vi "Test MinMax Decimation.vi"() -> ()   [LabVIEW 2020, in "VolatusScratch.lvlib"]
uses:
  VolatusScratch.lvlib
  VolatusGUIElements/VolatusGUIElements.lvlib
  <vilib>/Analysis/NI_AALBase.lvlib
panel:
  in  "Width":dbl=20.0 format="%#_13g"
  in  "Length s":dbl=10.0 format="%#_13g"
  out "XY Graph":cluster{dbl[], "Sinusoidal Pattern":dbl[]}[](graph)
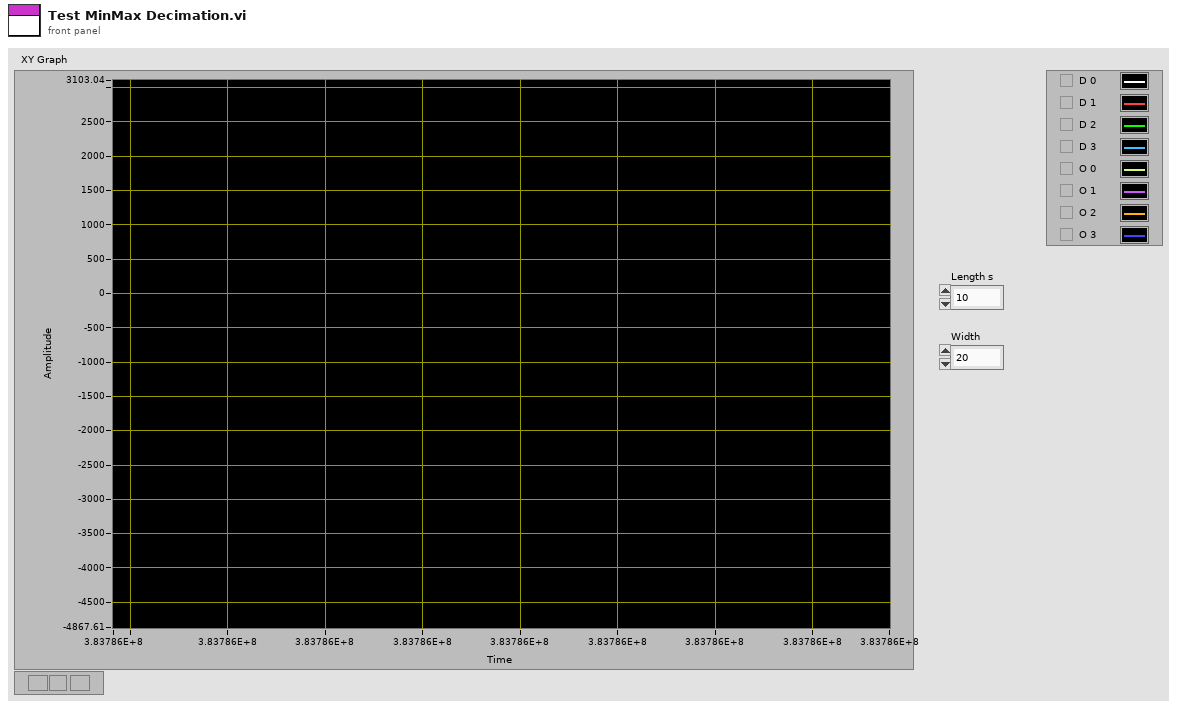
[diagram p1: front panel]
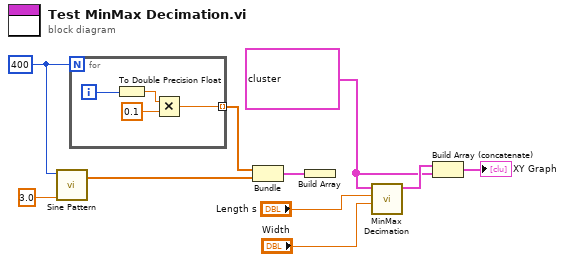
[diagram p0: block diagram]
diagram:
  w1 = cluster{dbl[], "Sinusoidal Pattern":dbl[]}[] [{array[5416 elements], "Sinusoidal Pattern"=array[5416 elements]}, {array[5416 elements], "Sinusoidal Pattern"=array[5416 elements]}, {array[5416 elements], "Sinusoidal Pattern"=array[5416 elements]}, {array[5416 elements], "Sinusoidal Pattern"=array[5416 elements]}] ("appended array")
  w7 = 400 ("samples")
  n1 = call <vilib>:"Sine Pattern.vi"("cycles"=3.0, "samples"=w7) -> ("Sinusoidal Pattern"=w6:dbl[])  [unwired: 2 in, 1 out]
  n2 = for {
    N: w7 -> [_]
    tunnel: [w11] -> w5 mode=indexing
    i -> [w14]
    n3 = To Double Precision Float(number=w14) -> (double precision float=w13:dbl)
    n4 = Multiply(x=w13, y=0.1) -> (x*y=w11:dbl)
  }
  n5 = Bundle(w5, "Sinusoidal Pattern"=w6) -> (w4:cluster{dbl[], "Sinusoidal Pattern":dbl[]})  [unwired: 1 in]
  n6 = Build Array(w4) -> ()  [unwired: 1 out]
  n7 = call "MinMax Decimation.vi"("Width"="Width", "Length s"="Length s", "XY Data"=w1) -> ("MinMax Data"=w3:cluster{dbl[], dbl[]}[])  [unwired: 8 in]
  n8 = Build Array (concatenate)(w3, w1) -> (→"XY Graph":cluster{dbl[], "Sinusoidal Pattern":dbl[]}[])
